vi "SUB_NICARD_DTMF9.vi"(3 "Time Out 秒":dbl, 4 "需找到特定KEY被壓的次數":i32, 5 "Find this char":string="9", 6 "AI_Name_Receiving":string) -> (0 "Detected Numbers":string, 1 "Total Count":i32, 2 "Pass?":bool)   [LabVIEW 2011]
doc: "This example shows how to construct a simple Spectrum Analyzer example using the EASY I/O Sound VIs and the MEASUREMENT VIs. This example acquires a waveform, windows it, computes the autopower spectrum and the power and frequency of the peak frequency component. The power spectrum is graphed in the desired units."
uses:
  <vilib>/sound/lvsound.llb/Sound Format.ctl
  <vilib>/DAQmx/configure/timing.llb/DAQmx Timing (Sample Clock).vi
  <vilib>/DAQmx/create/channels.llb/DAQmx Create Channel (AI-Voltage-Basic).vi
  <vilib>/DAQmx/read.llb/DAQmx Read (Analog 1D DBL 1Chan NSamp).vi
  <vilib>/Analysis/NI_AALPro.lvlib
panel:
  out "error out":errorcluster
  out "Begin Time":u32
  in  "clear":bool
  out "high tone":dbl
  out "low tone":dbl
  out "Spectrum Plot":cluster{dbl, "df":dbl, "Spectrum out":dbl[]}(graph)={0.0, "df"=10.7666015625, "Spectrum out"=[2.2239345811923915e-09, 8.683146662335903e-05, 5.401658948819699e-09, 3.283415769949573e-09, 9.087470257203412e-09, 5.196356826384313e-09, 1.0843872733561082e-08, 4.3666839571391997e-08, 7.323773949015906e-09, 2.8497866290202407e-08, 1.8346139778676557e-08, 8.325138799005256e-08, 3.709426329648907e-07, 1.0144554155621068e-07, 1.4859985315839882e-08, 2.4076563517443918e-08, 1.3199122618695927e-08, 3.4089918312362413e-07, 3.6647748653227776e-08, 2.1872311499262826e-07, 8.686470585259585e-07, 1.3633533191204446e-06, 1.809178172260895e-06, 6.207150699649024e-07, 1.88584897213167e-06, 9.53443075462152e-07, 8.595628778203373e-06, 1.6534093489189502e-05, 8.565381366748433e-06, 3.934368638186503e-06, 2.673398134714082e-06, 7.620166221013746e-07, 2.018558207269129e-06, 2.445724570769696e-05, 4.90872869304964e-06, 1.2172709001598665e-05, 9.405478455395956e-06, 1.6026544209442022e-05, 3.1157695023137614e-05, 0.00010045066273845566, 0.00010099562444668703, 0.00010789070486165799, 1.915813665106557e-05, 1.0487977511963416e-05, 7.094885886145816e-05, 3.322502717803691e-05, 3.175752599123204e-06, 6.984547958898752e-06, 8.122003278929465e-05, 7.657590620424026e-05, 6.720711760531132e-05, 0.00027943324712291083, 1.9805707230316307e-05, 4.50827477517238e-05, 6.0571130135876217e-05, 0.00021856285906605584, 0.00038709341896675954, 0.0002252713059067297, 0.00013722927061328232, 0.00025744130739904097, 0.00031585831536121644, 0.00028812421894327536, 8.629231121040524e-05, 0.00019142781529715328, 0.0017885090818483191, 0.004444937101978304, 0.002747724841296513, 0.00011579632868297775, 0.0013646075587948122, 0.0035542620245009146, 0.001429284269391688, 4.9135884119093836e-05, 0.00010438991046028727, 0.0002092766335322915, 0.0005706029316243163, 0.0011927099686592443, 0.002202098299693849, 0.0042447756964313806, 0.002184938955182395, 0.0013931881329623834, 0.000611791345491331, 0.00014384098592416903, 0.002089648172238157, 0.0014604892491541625, 0.001672902813259857, 0.0020996846985977796, 0.0018267042820125684, 0.00024143153807025544, 0.002728954825480649, 0.00016124193611955143, 0.007491288639908926, 0.01608076261438152, 0.0076505026127518016, 0.0009127306549049931, 0.00011906946681760085, 0.0006340416871388245, 0.0007338175758111943, 2.5182502508708624e-06, 0.0014774150320969704, 0.0034280107997651014, 0.004065940033575572, 0.0001807139654879104, 0.0015134026443213385, 0.0011456998362453944, 0.00010824998720249853, 0.002948833243774608, 0.00012048947131529409, 0.0032335488260886737, 0.003226548109806722, 4.90267994721965e-05, 0.00069147886170929, 5.666823215140518e-05, 0.0005823192819762041, 0.0009022477028271505, 0.0005517533787869191, 0.0003117207285129016, 0.0003908753871750581, 0.0001541062450876749, 0.00039676777157499044, 0.00021195970391491326, 2.6234631508778257e-05, 0.0002658837847014447, 0.00036345197596954665, 0.0003636016946459504, 0.0002883525548514524, 0.0002323997797870554, 0.00045117546603606835, 0.0007831715089129511, 0.00037697969403779224, 0.00025684169148288533, 0.00010464265607880238, 0.00015392030920770804, 0.000571268118545142, 0.0001791281135008112, 1.82407915272795e-05, 1.3435216977496377e-05, 6.613286083519268e-05, 6.85306300694302e-05, 3.106260409346511e-05, 7.043306599712916e-05, 7.446350251160272e-05, 7.807453839697811e-05, 4.641495088994314e-05, 4.594124976757755e-06, 2.6361087556609282e-05, 5.408410897184997e-05, 4.840864204869872e-05, 3.0852881930333154e-05, 1.4632960335315108e-05, 7.27125525658015e-05, 0.0001295923092952229, 8.06079297415985e-05, 1.2892262186773693e-05, 3.912635943158275e-05, 0.00018875463470383673, 0.00046239539279871813, 9.83461014422302e-05, 0.00010431991121427508, 5.7426568744302205e-05, 1.2919647585699225e-05, 1.3333446843951983e-05, 8.00557455545567e-05, 0.0002140654846038062, 0.00018799784777159107, 8.297670421251171e-05, 3.356795673514294e-05, 9.249862040099823e-06, 2.9018278924853506e-07, 4.5754135907992884e-05, 5.226444686010533e-05, 1.3393528265419317e-05, 5.861689249679998e-06, 6.754517491150961e-05, 0.00025201542605521695, 0.00012663622684922263, 8.354734534008234e-05, 9.900401690907939e-05, 1.0203246067824091e-05, 1.3846422437959727e-05, 1.7513782918600468e-05, 2.2531470225547707e-05, 3.570026999460579e-05, 5.608394459352944e-06, 3.5507984663188685e-08, 6.193650127282948e-06, 5.485683901026815e-06, 4.893254891786411e-05, 5.752391322110518e-05, 3.500417190819705e-05, 3.491426035627687e-05, 1.2227919637292493e-05, 9.326738918780702e-05, 0.00012903483454479285, 0.00011419716448848833, 8.886505769204026e-05, 2.9281175535596163e-05, 8.132081786205703e-06, 8.97985862152433e-07, 4.8247392248735155e-05, 5.367945684187481e-05, 3.633225820245703e-05, 9.022031345501884e-06, 2.0929305851300513e-05, 6.752089148961767e-06, 3.286214637706205e-06, 3.6662630198477625e-07, 7.763291731476242e-07, 1.3399945907103394e-06, 5.085966555258911e-06, 1.077887668545493e-05, 1.1281582963565783e-05, 1.155397820681578e-05, 4.6520974337610276e-05, 2.3309391421773472e-05, 6.845693658632664e-06, 2.704122544346558e-06, 6.665125665645291e-06, 1.0876441922754335e-05, 5.608797346818875e-06, 8.296695137818328e-07, 2.03813752326054e-06, 1.0973914063981042e-05, 1.9892910350080524e-05, 4.191121605107763e-06, 1.808715991023127e-06, 9.795606447014282e-06, 9.022632252180524e-06, 2.2366113182871527e-06, 1.436223524998135e-05, 5.7260934078321705e-06, 4.825080996478945e-06, 2.1388562191637884e-05, 1.763101781807734e-05, 2.2587628529471817e-06, 1.983067720399453e-07, 3.909338538260015e-07, 4.5350273020466913e-07, 8.343654577854134e-06, 6.790839886647775e-06, 2.255636327297339e-06, 2.584488445117655e-06, 6.824174854821624e-08, 1.372661787015302e-06, 7.194056251356914e-06, 4.541157254321738e-06, 1.6303668540732263e-06, 8.110116936046172e-07, 9.818519159870482e-07, 6.537064705721577e-07, 6.165130865665045e-07, 6.814246977481835e-07, 5.142784956191243e-06, 1.2862670435653503e-06, 3.431212791692102e-06, 6.717152893884229e-07, 5.0793672092905424e-06, 5.091843002358143e-06, 3.3788601899426006e-06, 1.6294942179365793e-06, 3.2052888551651294e-06, 2.505011537891627e-06, 1.8986099392174936e-06, 8.895175541066118e-07, 1.3175069598051258e-06, 4.119412961373611e-06, 1.7694268293659887e-06, 4.6245139735427074e-07, 4.085574744081603e-06, 6.641800395694785e-06, 2.3866053854954935e-07, 6.7501963295773596e-06, 1.3861042484181615e-05, 3.691970172195625e-06, 3.9272846697908543e-07, 3.1694989865639504e-07, 2.201281939330297e-06, 1.9502880819500733e-06, 9.578342900676284e-07, 3.83131360027214e-08, 1.9515784635010561e-07, 2.9878004194019836e-06, 4.081752511669434e-06, 7.209641153264918e-07, 8.693458519441707e-08, 4.6824501323622113e-08, 1.6560973862183618e-07, 2.0079696309823287e-07, 2.1630743971307335e-06, 2.23361594841029e-06, 3.166336475982508e-08, 1.419563103629219e-06, 3.0006577783992975e-06, 2.124654816469341e-06, 4.1221962384799796e-07, 1.4312683542199081e-06, 1.7737127563135207e-06, 9.697151883610893e-07, 7.954478190626394e-07, 1.1992527144472837e-06, 8.855607963063999e-07, 1.6461066449965424e-07, 1.7397212300863859e-07, 8.556536030808307e-07, 1.353353790123818e-07, 9.394460603994867e-07, 1.4424479309137508e-07, 1.6772776914222815e-07, 7.247702472793038e-07, 1.9063669000254936e-06, 1.887443849495326e-06, 1.8925707210222315e-06, 1.0040375911083587e-06, 7.552902303940092e-07, 1.8020303869132393e-06, 1.0587142496314781e-06, 1.459031411847178e-06, 1.4347870788937637e-06, 2.0172474849463537e-06, 1.516022898250378e-06, 3.2596374238585613e-07, 2.1549499015163616e-07, 2.586117511547747e-06, 1.8362715158444338e-06, 1.3581697014034016e-06, 9.715110917820086e-07, 2.2519613957274757e-08, 8.046610762626154e-07, 1.1130490891085315e-06, 1.3216986457543798e-07, 8.016611790474239e-07, 7.954966525566603e-07, 3.287552824052373e-07, 3.1999251102532676e-07, 1.9773782303361322e-06, 7.57049324561171e-07, 2.899671781808912e-07, 1.9745982550542387e-06, 1.4817821073364632e-06, 4.2207281783042705e-07, 2.859510597989451e-06, 6.65169327673545e-07, 1.3108579688597603e-06, 1.9279525632742265e-06, 1.923607859494516e-06, 3.7608877809167786e-07, 8.770605149941596e-08, 1.4085300538439131e-06, 1.2665811768763722e-06, 1.8672220783028666e-07, 1.6249157461690274e-06, 3.0133475481236383e-07, 6.955888433270435e-07, 1.4486995359594106e-06, 1.19907829055927e-06, 9.753115535094555e-07, 4.6454715494736343e-07, 2.454857073207436e-06, 5.444677191663221e-06, 3.151266111199155e-06, 2.0365010021356476e-06, 3.763692357617005e-07, 2.8048385043293254e-07, 7.267621498153388e-07, 1.897445548683447e-06, 9.801545193276826e-07, 5.034122710723187e-07, 8.546959157775001e-07, 5.726282029332936e-08, 1.790518893028658e-07, 1.619379081284686e-07, 1.6374366581195436e-06, 2.2925538126773367e-06, 4.1761747260056753e-07, 3.958797175774531e-07, 7.972425726207277e-07, 3.4033204403124756e-07, 1.940413284776906e-06, 7.47966836993988e-08, 1.4378795743103673e-06, 8.471793410934394e-07, 4.6447241003195404e-07, 1.6666364624086332e-07, 6.184453795459414e-08, 1.038190704797001e-07, 6.865153388263582e-07, 5.491932744056226e-07, 7.736989677920619e-08, 4.874378562302079e-07, 3.00965029667906e-07, 5.423676481238429e-07, 6.72738762673129e-07, 5.018387553252361e-07, 1.4247024148982255e-06, 3.4300270666082203e-07, 1.6301756163139806e-06, 1.8215300880149825e-06, 1.0797103355618773e-07, 1.9041653191023335e-07, 7.743539027667847e-07, 4.534623961465652e-07, 2.2330057360512448e-07, 3.132811548231781e-07, 1.022133188486526e-06, 6.274155220759265e-07, 6.903427238780778e-07, 7.33567481947441e-07, 2.047023910845942e-07, 2.791277398928224e-07, 1.3222939038823352e-06, 1.2382074249353341e-06, 3.0602357137379264e-08, 3.226519226595554e-07, 1.4358933700160236e-07, 2.161999598210508e-07, 7.226405438923372e-07, 7.82781403633883e-07, 1.406298955204302e-06, 1.2978368125295453e-06, 1.0787385566291683e-06, 7.74693414922409e-07, 1.0280376744316506e-07, 1.897257118504827e-07, 4.0674154164735285e-07, 3.3330924842068594e-07, 5.647220323383419e-07, 1.3067977141464316e-07, 6.21291802684579e-08, 6.959387220834736e-08, 2.978875001494869e-08, 1.1417698207989842e-08, 1.1088891892277042e-06, 2.1693278042962233e-06, 1.3106423009701006e-06, 9.751035000237095e-07, 3.9079154946663974e-07, 1.9665634688411184e-07, 8.019395828747413e-08, 5.648358376218229e-07, 8.755518865790549e-07, 2.1544487475681563e-07, 8.997104969411794e-08, 2.6406756196946574e-07, 9.499330882404733e-07, 4.6505226539756276e-07, 1.683265150296703e-07, 1.9973962216810128e-07, 4.5604784891804473e-07, 1.0038766206556954e-07, 1.2139267125159811e-08, 3.600082456137448e-08, 6.456671217308024e-08, 4.5206944177849573e-08, 5.120895166543777e-07, 5.020703551538299e-07, 1.4358445110590547e-08, 1.087422035023867e-07, 2.904937040652121e-07, 9.965912368812135e-08, 1.567195405704097e-07, 3.607977162533612e-07, 8.661286097636492e-07, 2.0043494023967716e-07, 1.404349876871561e-08, 1.155747877697829e-08, 8.948817141186363e-08, 5.8027285180593554e-08, 4.073116484984666e-08, 1.3308592777960855e-07, 2.3957183564679474e-08, 6.957435335895439e-08, 6.155244039483246e-08, 2.4444043310448568e-08, 2.670800778057559e-08, 5.7216353702400666e-08, 9.239854415332251e-08, 3.0213042230580236e-08, 1.343191141960498e-09, 2.0837817399160295e-08, 2.602661931976853e-08, 6.8560172643748795e-09, 7.916856835570337e-08, 9.00267241744782e-08, 7.692528448413547e-08, 1.2004889715129119e-08, 9.88727747790812e-08, 1.0023405452613187e-07, 1.210633991600998e-07, 2.1522628537105935e-08, 5.6078990716154034e-08, 5.4328268985728565e-08, 7.382864407910501e-08, 3.0003386035033976e-08, 1.2666181215774758e-07, 1.447357694076088e-08, 4.5027939045110415e-08, 5.3269947199899464e-08, 3.859299030969913e-08, 3.241786088144045e-08, 2.720065882503426e-09, 1.2643450599208627e-08, 1.964613447417824e-07, 2.0620303225395736e-07, 3.960659464702874e-08, 5.470531246980156e-08, 2.1669113140794644e-08, 3.908095826759173e-09, 2.49346348700968e-09, 6.457620819587205e-08, 7.514895182622606e-08, 9.756339699497464e-09, 6.350841154899524e-09, 1.2441504257846113e-07, 2.140824153645837e-07, 7.93683699567381e-08, 2.9681442249265694e-08, 1.0955395323608218e-08, 4.758727775105736e-08, 3.1114217067159584e-08, 2.8431649831268218e-08, 7.886529468547796e-08, 6.928095914063998e-08, 6.44062797559934e-08, 1.5729337740057154e-07, 1.633584064839165e-07, 3.805955578821095e-08, 3.4997453344192845e-08, 8.022151382112027e-08, 8.574249753493645e-08, 8.12990606975002e-08, 1.9694836264953252e-08, 1.0791818303309123e-08, 1.570533231452924e-08, 7.382425248896943e-10, 3.9250377730515e-08, 4.72955171147271e-08, 8.090028033459793e-08, 1.0325474748498492e-07, 5.1119681074873145e-08, 7.094343264085443e-08, 2.9392859253071123e-08, 9.238628151896506e-09, 5.694530625648633e-08, 1.8625727600349932e-07, 3.322703462873384e-08, 3.425440210880957e-08, 3.4277236525869975e-08, 3.617970164543665e-08, 1.4707673577394132e-08, 1.2922454182753588e-10, 1.8095931082295038e-08, 5.600407565406485e-09, 8.953513148727372e-09, 2.3611851256797674e-08, 1.146166540157641e-08, 2.201964779928675e-08, 2.9764039172426437e-08, 2.961234359885526e-08, 5.5575454720846034e-08, 1.590716964180081e-08, 2.5499378001220853e-08, 8.486556471190526e-09, 4.204027722433145e-09, 1.0654218030939125e-08, 5.474455330294607e-08, 5.4653270431217174e-08, 4.783079993275118e-08, 4.6046354336983404e-08, 7.990893299542365e-09, 2.3198558294294397e-08, 2.9547812456393353e-08, 1.2653880062427829e-08, 1.7251579240159026e-08, 4.63416262611152e-08, 1.5129601159503794e-08, 2.3139266486687776e-09, 1.828690977536453e-08, 2.2861672881711013e-08, 3.8144074954067966e-08, 2.8840406985371016e-08, 1.1468655141246242e-08, 1.6179157979919108e-08, 2.9612534185614193e-08, 4.232564980227527e-08, 5.807228261326083e-09, 1.193918664246388e-08, 9.555146125407209e-09, 2.6756709498907878e-08, 3.5854514290437304e-08, 3.3536922761277736e-08, 1.6236282954676824e-08, 1.419182533462672e-08, 1.8960043424887072e-08, 2.2529888699703793e-08, 2.769640618611182e-08, 1.7752768144773262e-08, 3.817051129247205e-08, 3.9146068301267074e-08, 2.701166800566469e-08, 3.6083532480292083e-08, 4.759826701599105e-08, 2.2528709606772587e-08, 1.4373847425932876e-08, 1.0108916334457278e-08, 4.344209392987958e-09, 2.76248817252588e-09, 3.345855814497143e-08, 3.1876958273761295e-08, 1.0309771452695787e-08, 7.480054719232873e-09, 6.934965945389653e-09, 1.021958155170289e-08, 4.726637225820998e-09, 2.7923791885579298e-08, 2.615594662610562e-09, 5.685726703733775e-10, 6.436791353396253e-09, 3.971859921789547e-09, 5.451134199864811e-09, 5.599761079275237e-09, 1.8091294273463573e-09, 6.459132929182603e-09, 5.657936238218396e-09, 1.950038474358936e-08, 3.902896651024208e-08, 2.6647511591608208e-08, 1.7167991854833567e-08, 5.705082172612073e-09, 1.1906878405088487e-09, 6.430332981144355e-10, 3.044261872785727e-10, 5.40091869318323e-09, 1.145469490858611e-08, 4.512515382960901e-09, 1.268872354479999e-09, 8.69571281338811e-11, 5.979719362973721e-09, 8.303067196362185e-09, 1.039890454681567e-09, 4.403612351010871e-09, 6.1893486406988e-09, 3.744143658237287e-09, 1.6098151770992428e-09, 5.248990067906987e-10, 8.470755606628997e-09, 7.463249915147587e-09, 1.0295767797537241e-09, 3.4956972619547825e-09, 5.641606872154712e-09, 4.994213570996723e-10, 2.405446245720403e-09, 1.489678532464873e-09, 2.2902032474967982e-10, 1.8935576252770074e-09, 6.140797401991911e-09, 4.138757232522736e-09, 1.4205243196923323e-08, 1.0122644492215224e-08, 1.0308696632691912e-09, 3.7261704680704176e-09, 2.219667711519674e-09, 1.5818367931203758e-10, 3.1956703588648097e-10, 3.728028330933628e-09, 5.204819070783557e-09, 2.3182128777113778e-09, 5.54274237431268e-09, 5.912467923961738e-09, 3.4984304800838524e-10, 1.7519583360697777e-09, 3.5760658885376834e-09, 2.920707192498906e-09, 4.991604442354138e-09, 5.22047326033885e-09, 1.1121882980094295e-08, 1.0515997862901546e-08, 8.56222533176954e-09, 2.16240545488912e-09, 3.4438501798671816e-10, 1.8304744483799816e-09, 7.928375487876729e-09, 5.625674085292935e-09, 2.599916438756517e-09, 3.5181591731768393e-09, 2.1217829342968287e-09, 2.2753003599648508e-09, 3.4226665411631988e-09, 5.636839365927383e-09, 7.482358015828702e-09, 3.4894051216861324e-09, 5.081541309898216e-10, 5.232121738196756e-10, 3.4140952661333457e-09, 5.535791400541489e-09, 2.330868115515569e-09, 7.282566020209013e-10, 7.872180714469127e-10, 2.0937186224820734e-09, 4.385762477016771e-09, 4.662321859562959e-09, 1.0936849727646788e-09, 1.779919440059085e-09, 5.814676588780071e-10, 1.4243028963503696e-09, 7.711594786984741e-09, 3.529621264712184e-09, 2.676389419868003e-09, 4.024900708447496e-09, 8.979532033775118e-10, 1.387096810631821e-09, 6.16168707641335e-10, 1.3043500724006639e-09, 1.0060661688154498e-09, 5.272350241092032e-10, 4.842385157592935e-10, 4.79401273594476e-09, 5.555714769211231e-09, 3.071678971190096e-09, 4.256573526238938e-09, 1.928446419086416e-09, 4.416159046828467e-10, 3.767639009725344e-09, 2.952303872960992e-09, 1.7643182268094367e-09, 1.184159894053597e-09, 2.7932934526917684e-09, 1.9368817963660564e-09, 2.7430528754171613e-09, 5.225587432169088e-10, 3.203199932968183e-10, 1.9797615162730513e-09, 8.560689437790192e-10, 1.3756570831157762e-09, 2.077805905489259e-09, 3.53465334234968e-09, 4.860234675895279e-09, 2.124017257302096e-09, 5.853203456602198e-11, 2.516050984534377e-09, 7.880997614550843e-10, 7.37630554137802e-10, 7.31937655708805e-10, 7.602633332778057e-10, 1.4973872311600496e-10, 2.832501177732104e-09, 3.4088527208373545e-09, 2.10419737941665e-09, 1.7856704137105817e-09, 1.8829909904485974e-09, 1.6885012672101362e-11, 9.981932083310103e-11, 4.923391793317421e-10, 5.488431723286112e-10, 3.1535776708464555e-11, 1.2576645527152945e-10, 3.195193563516089e-11, 2.9010054595514423e-11, 5.3959324436706067e-11, 4.207578635912359e-10, 1.3434752942557352e-09, 8.388553690154514e-10, 3.709413955497562e-10, 2.310126954666965e-11, 1.9412886393254603e-10, 1.5256275616250847e-09, 1.2700530378170274e-09, 1.0145820142699707e-09, 9.02812894090267e-11, 2.380865008764687e-10, 1.3884639791549605e-10, 7.097231542592393e-10, 1.4705312317889802e-10, 3.862728542670797e-10, 6.164191610984895e-10, 2.660938261830858e-10, 4.1980202338370243e-10, 4.174891700935234e-10, 1.9551068467012963e-10, 1.2809251895251019e-09, 1.2010818631768713e-09, 8.023763127102151e-10, 2.301277278510448e-10, 2.282367771403777e-10, 2.802656534310578e-10, 2.8381567604717416e-09, 1.3056140440628833e-09, 9.946000302107385e-10, 2.019650934949039e-10, 6.17402391077043e-11, 5.067315270594634e-10, 8.495763773619358e-11, 7.685765214095721e-12, 6.596099326938714e-11, 1.5977878807757865e-10, 1.3505898652283798e-10, 3.2339161959433536e-10, 9.181248445894812e-10, 9.033526336502124e-10, 9.365426508084887e-11, 1.5835643049796864e-09, 1.109253745919973e-09, 4.743298781860182e-10, 3.987212410725e-12, 9.016453427310602e-11, 2.2564563875148533e-10, 2.170213485823025e-10, 2.4632504239019264e-11, 8.685537809384159e-10, 5.0716890250874e-10, 8.171582894823122e-13, 1.2319527875084226e-10, 2.794878076018828e-10, 1.9098550224368597e-10, 2.243856772517594e-10, 3.721139454800636e-10, 7.543450869519107e-11, 5.492907359358165e-10, 7.441572939818098e-10, 5.563714854922252e-10, 2.3442621156495966e-10, 7.122534088655344e-12, 5.438935026364515e-11, 3.058752272772633e-11, 7.964657206284309e-11, 1.322930734820325e-10, 4.1828035722374734e-10, 4.825514587076015e-10, 2.3601908260282152e-11, 9.995037669671284e-11, 2.8837286106756752e-11, 7.7584161635509e-11, 4.925186582086759e-11, 4.3123223628482706e-11, 6.001348439876205e-11, 2.660823203179512e-10, 5.835097679116502e-11, 2.4371074101681597e-12, 2.8708263655531525e-10, 1.0452331220034235e-10, 1.7419411308588767e-11, 1.586938787690648e-11, 2.614011077415245e-10, 1.906391801272774e-10, 8.608172097402236e-10, 6.359406235781075e-10, 9.55087274351948e-11, 7.420039646561873e-10, 4.277854440466337e-10, 2.514884199120615e-10, 1.87362909024348e-10, 5.816583664209649e-12, 3.0748210371688494e-11, 1.1617001225093083e-10, 1.543372698055287e-10, 2.1164907244552623e-11, 1.5339034521507372e-10, 1.1296774574948826e-10, 3.545703672449203e-10, 6.838348267836377e-11, 2.666691344937961e-10, 4.01146646127394e-12, 2.8253853309552043e-11, 4.865860582627764e-11, 3.812971990283942e-11, 3.513905009113374e-10, 7.262049749655285e-11, 2.7076218803863766e-10, 1.679038424025831e-10, 1.191512488410735e-10, 1.6762637771545003e-10, 1.1570677133729292e-10, 2.93701692757346e-11, 8.985694145300448e-11, 5.378560526480976e-12, 1.5111522532685182e-11, 9.33784088613121e-12, 8.108969569702798e-11, 7.344604239441166e-11, 2.749158285282731e-11, 1.149440726370342e-10, 7.558184550049066e-11, 1.0388688445068887e-10, 2.3884411611108205e-11, 4.523702881859529e-11, 5.539444652117604e-11, 1.2505846602408144e-10, 1.391237889983128e-10, 1.0229838641777619e-10, 2.2760448461751894e-10, 1.6878930272235683e-11, 5.563133519338542e-11, 2.4795564168072182e-11, 4.88300841319007e-12, 2.753076326726938e-10, 5.0745585442639115e-11, 1.9748881750443707e-11, 4.7253681970740655e-11, 1.1828022584495795e-12, 6.307397956109176e-11, 1.2112903811280616e-11, 3.7736829220246094e-11, 1.2666717771535954e-11, 9.110131621536755e-12, 1.4356147174808164e-10, 4.835735472117299e-11, 1.6119503703271416e-10, 2.7284220732102933e-11, 6.252917322874483e-11, 4.3224534315473703e-11, 1.0498695216758215e-10, 1.974346778432821e-11, 5.40782337396056e-11, 5.2369100478518394e-11, 2.2326679398260537e-12, 1.3443392922630235e-10, 1.5137082145318955e-11, 7.602967117655898e-11, 1.6705324428778388e-12, 8.087034464306943e-11, 2.843203593917431e-11, 4.3869855642256153e-11, 9.094608127233439e-12, 5.1610906648717704e-11, 4.5769346158818275e-11, 8.91014346500043e-12, 2.1390251716311653e-11, 6.369147522118072e-11, 2.0219657267618414e-11, 7.614932077706351e-11, 8.380130770612789e-14, 7.44685721218674e-11, 4.889713918700368e-12, 2.8824435687798222e-11, 2.336178035548185e-11, 2.032069895529248e-11, 3.177186397825414e-11, 1.829839515856845e-11, 1.7199587674909958e-11, 2.3830341916764486e-11, 3.936674241530467e-11, 1.4530112344764962e-11, 6.42340167219902e-11, 6.543850560478522e-12, 3.180552492573337e-11, 2.640733156400162e-11, 2.3998816474733135e-11, 1.4707500600098032e-11, 2.2677492907918244e-11, 2.5488024985826562e-11, 2.2847423539048195e-11, 2.6508742451231927e-11, 2.7455219413636878e-11, 1.9014114797814238e-11, 1.4498235090545703e-11, 2.971065931438831e-11, 2.8238743649172455e-11, 1.5558166743438014e-11, 1.5480415800015573e-11, 2.743925897718036e-11, 2.7495492280695883e-11, 9.799113867949333e-12, 3.6747692894834385e-11, 8.199934716177243e-12, 4.0755373799372346e-11, 2.121428785076837e-11, 1.5541949260482237e-11, 2.798920514032833e-11, 1.7462178669667912e-11, 2.344077180370279e-11, 1.3268735286972787e-11, 3.290786429192333e-11, 1.3582414980189854e-11, 2.1254639689841874e-11, 3.125190775410135e-11, 1.1594584974728011e-11, 2.0766725629006086e-11, 2.5397224688363225e-11, 2.017197976315566e-11, 2.1560267022375116e-11, 1.8478426377320472e-11, 2.185880297981598e-11, 2.3207271921244853e-11, 1.6644091551449067e-11, 2.5159531873055792e-11, 1.7387326911492145e-11, 2.2342088396302478e-11, 1.878186953930171e-11, 2.1386854408980777e-11, 1.6296384472522648e-11, 2.665785605014739e-11, 1.932225503661904e-11, 1.7990103900180257e-11, 2.280409760981406e-11, 2.0876076757621922e-11, 1.6705840903949015e-11, 2.447838243286913e-11, 1.9386127278251222e-11, 1.9972810505022722e-11, 2.094081228451663e-11, 2.089112317638976e-11, 1.8529128535041152e-11, 2.1003285317481698e-11, 2.1626975006946126e-11, 1.959173405923362e-11, 1.9951310126412882e-11, 2.056616361421096e-11, 2.0129355353149965e-11, 2.081460915369522e-11, 1.9548428298641114e-11, 2.099219771829391e-11, 1.969977451051827e-11, 2.0914920833116317e-11, 1.976452612506575e-11, 2.061186299405415e-11, 1.994600938714932e-11, 2.0573926789305875e-11, 1.9999209922834507e-11, 2.0465454689399724e-11, 2.0178494817701738e-11, 2.0384946662937728e-11, 2.0181301433592506e-11, 2.0287338520900114e-11, 2.028072242449754e-11, 2.0263007390114753e-11, 2.0273179004249868e-11]}
  # "Settings"
  # "Detected Tones"
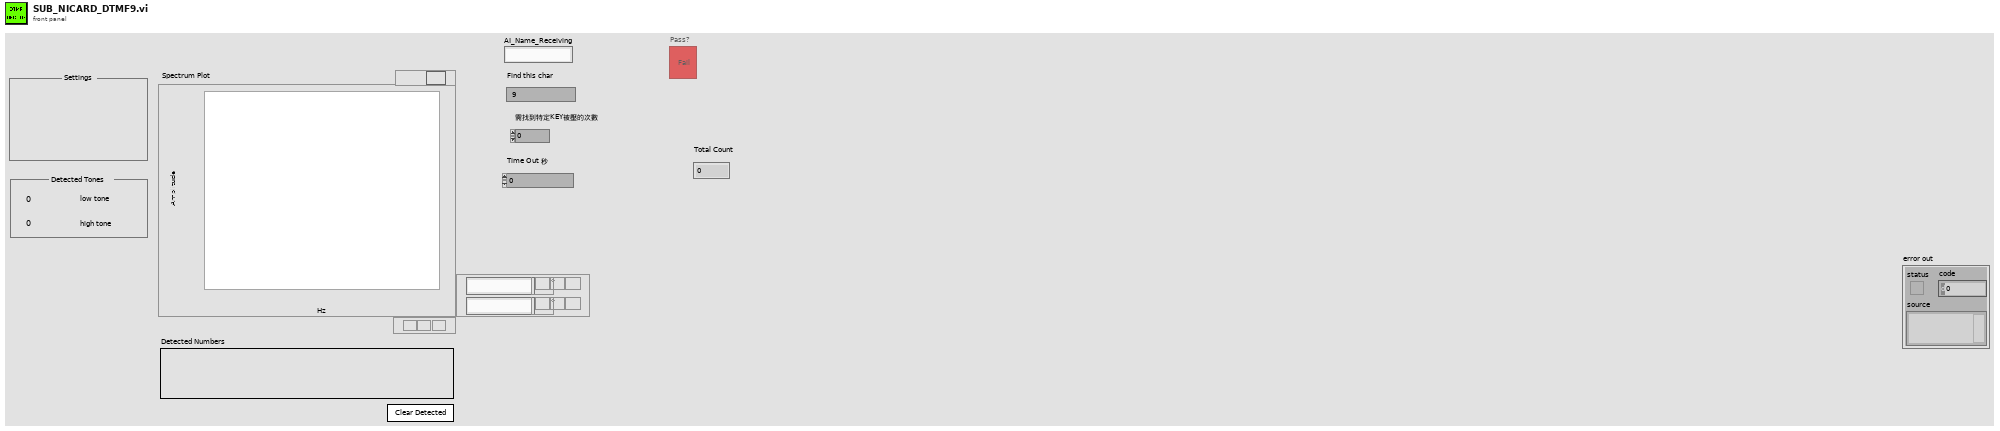
[diagram p1: front panel]
types:
  T1 = typedef "Sound Format.ctl" = cluster{"sound quality":enum16{"mono", "stereo"}, "rate":enum16{"11025", "22050", "44100", "8000"}, "bits per sample":enum16{"8 bit", "16 bit"}}
  T2 = enum32{"Lowpass", "Highpass", "Bandpass", "Bandstop"}
  T3 = cluster{dbl, "df":dbl, "Power Spectrum (V^2 rms)":dbl[]}
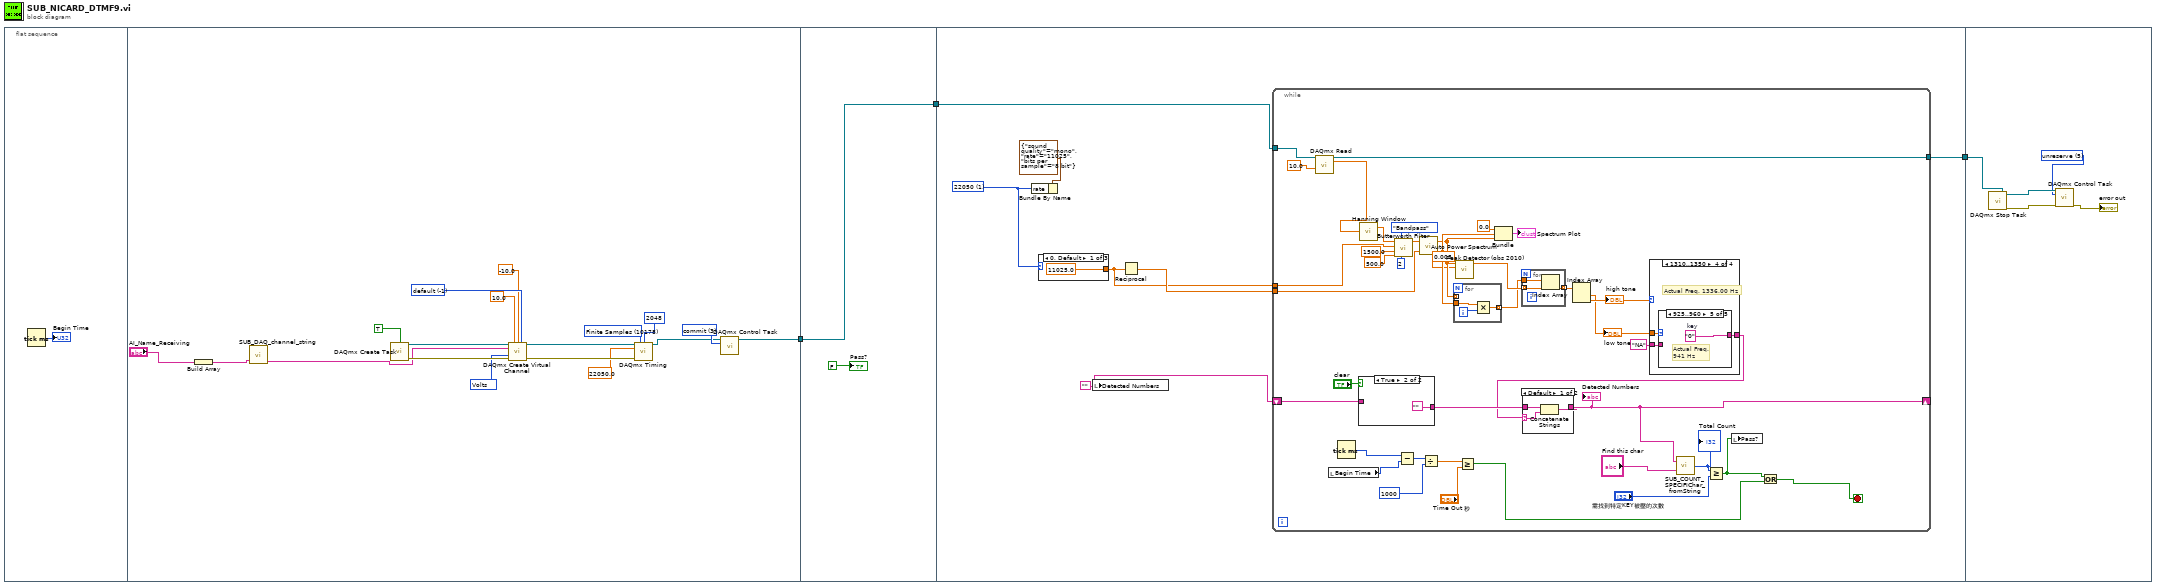
[diagram p0: block diagram]
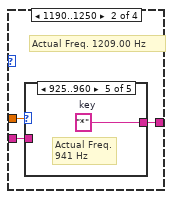
[diagram p5: hidden frame]
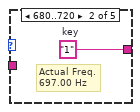
[diagram p7: hidden frame]
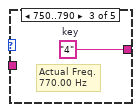
[diagram p8: hidden frame]
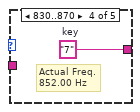
[diagram p9: hidden frame]
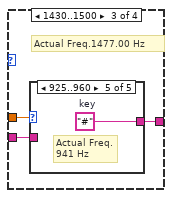
[diagram p10: hidden frame]
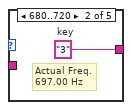
[diagram p12: hidden frame]
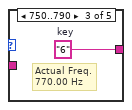
[diagram p13: hidden frame]
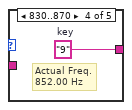
[diagram p14: hidden frame]
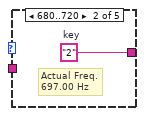
[diagram p16: hidden frame]
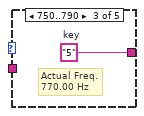
[diagram p17: hidden frame]
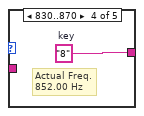
[diagram p18: hidden frame]
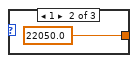
[diagram p19: hidden frame]
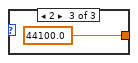
[diagram p20: hidden frame]
diagram:
  n1 = flat-sequence {
    tunnel: [w5] -> w2
    tunnel: [w23] -> w3
    tunnel: w2 -> [w23]
    tunnel: w3 -> [w26]
    tunnel: [w25] -> w1
    tunnel: w1 -> [w112]
    frame #0 {
      n2 = Tick Count (ms)() -> (millisecond timer value=→"Begin Time":u32)
    }
    frame #1 {
      w8 = -1 items=["default"=-1, "RSE"=10083, "NRSE"=10078, "Differential"=10106, "Pseudodifferential"=12529] ("input terminal configuration")
      w12 = 10348 items=["Volts"=10348, "From Custom Scale"=10065] ("units")
      w15 = 3 items=["verify"=2, "reserve"=4, "commit"=3, "unreserve"=5, "abort"=6] ("action")
      w17 = 10178 items=["Finite Samples"=10178, "Continuous Samples"=10123, "Hardware Timed Single Point"=12522] ("sample mode")
      n3 = Build Array("AI_Name_Receiving") -> (w9:string[])
      n4 = call "SUB_DAQ_channel_string.vi"("channel"=w9) -> ("resulting string"=w11:string)  [unwired: 1 in, 2 out]
      n5 = call <vilib>:"DAQmx Create Task.vi"("auto cleanup"=TRUE) -> ("task out"=w21:refnum<k21>, "error out"=w20:errorcluster)  [unwired: 13 in]
      n6 = call-poly <vilib>:"DAQmx Create Virtual Channel.vi"("task in"=w21, "maximum value"=10.0, "minimum value"=-10.0, "input terminal configuration"=w8, "physical channels"=w11, "units"=w12, "error in"=w20) -> ("task out"=w14:refnum<k21>, "error out"=w19:errorcluster)  [unwired: 7 in]
      n7 = call-poly <vilib>:"DAQmx Timing.vi"("task/channels in"=w14, "sample mode"=w17, "samples per channel"=2048, "rate"=22050.0, "error in"=w19) -> ("task out"=w13:refnum<k21>)  [unwired: 9 in, 1 out]
      n8 = call <vilib>:"DAQmx Control Task.vi"("task/channels in"=w13, "action"=w15) -> ("task out"=w5:refnum<k21>)  [unwired: 12 in, 1 out]
    }
    frame #2 {
      "Pass?" <- FALSE
    }
    frame #3 {
      w31 = u16 1 items=["11025", "22050", "44100"] ("Sample Rate")
      w27 = ""
      n9 = Bundle By Name(cluster=T1 {"sound quality"=enum."mono", "rate"=enum."11025", "bits per sample"=enum."8 bit"} ("sound format"), "rate"=w31) -> ()  [unwired: 1 out]
      n10 = case shown="0, Default" w31 {
        tunnel: [11025.0 22050.0 44100.0] -> w28
        frame 0, Default {
        }
        frame 1 {
        }
        frame 2 {
        }
      }
      n11 = local write "Detected Numbers"(w27) -> ()
      n12 = Reciprocal(x=w28) -> (1/x=w29:dbl)
      n13 = while {
        tunnel: w29 -> [w70]
        tunnel: w28 -> [w60]
        shift-right: [w48] -> _
        shift-left: w27 -> [w51]
        tunnel: w26 -> [w33]
        tunnel: [w32] -> w25
        stop <- w36 stop-if-true
        n14 = call-poly <vilib>:"DAQmx Read.vi"("task/channels in"=w33, "timeout"=10.0) -> ("task out"=w32:refnum<k21>, "data"=w34:dbl[])  [unwired: 11 in, 1 out]
        n15 = local read "Begin Time"() -> (w38:u32)
        n16 = Tick Count (ms)() -> (millisecond timer value=w37:u32)
        n17 = case shown="True" "clear" {
          tunnel: [w72 ""] -> w52
          tunnel: w51 -> [w72 _]
          frame False {
          }
          frame True {
          }
        }
        n18 = call "Hanning Window.vi"("X"=w34) -> ("Hanning {X}"=w61:dbl[])  [unwired: 1 out]
        n19 = call "Butterworth Filter.vi"("order"=2, "filter type"=T2."Bandpass", "low cutoff freq: fl"=500.0, "high cutoff freq: fh"=1500.0, "sampling freq: fs"=w60, "X"=w61) -> ("Filtered X"=w67:dbl[])  [unwired: 2 in, 1 out]
        n20 = Subtract(x=w37, y=w38) -> (x-y=w44:u32)
        n21 = call "Auto Power Spectrum.vi"("dt"=w70, "Signal (V)"=w67) -> ("df"=w56:dbl, "Power Spectrum (V^2 rms)"=w55:dbl[])
        n22 = Divide(x=w44, y=u32 1000) -> (x/y=w42:dbl)
        n23 = for {
          tunnel: w56 -> [w104]
          tunnel: [w103] -> w65 mode=indexing
          tunnel: w55 -> [_] mode=indexing
          i -> [w105]
          n24 = Multiply(x=w104, y=w105) -> (x*y=w103:dbl)
        }
        n25 = call <vilib>:"Peak Detector (obs 2010).vi"("threshold"=0.005 ("Detection Threshold"), "X"=w55) -> ("Locations"=w66:dbl[])  [unwired: 5 in, 4 out]
        n26 = Greater Or Equal?(x=w42, y="Time Out 秒") -> (x >= y?=w39:bool)
        n27 = Bundle(0.0, "df"=w56, "Power Spectrum (V^2 rms)"=w55) -> (→"Spectrum Plot":T3)  [unwired: 1 in]
        n28 = for {
          tunnel: w66 -> [w107] mode=indexing
          tunnel: w65 -> [w108]
          tunnel: [w106] -> w64 mode=indexing
          n29 = Index Array(array=w108, index=w107) -> (element=w106:dbl)
        }
        n30 = Index Array(array=w64) -> (element #1=w58:dbl, element #2=w59:dbl)  [unwired: 2 in]
        "low tone" <- w58
        "high tone" <- w59
        n31 = case shown="1310..1350" w59 {
          tunnel: w58 -> [_ w81 w89 w97]
          tunnel: [w78 w80 w88 w96] -> w49
          tunnel: "NA" ("Button") -> [w78 w79 w87 w95]
          frame Default {
          }
          frame 1190..1250 {
            # "Actual Freq. 1209.00 Hz"
            n32 = case shown="925..960" w81 {
              tunnel: [w82 w83 w84 w85 w86] -> w80
              tunnel: w79 -> [w82 _ _ _ _]
              frame Default {
              }
              frame 680..720 {
                w83 = "1"  # key
                # "Actual Freq. 697.00 Hz"
              }
              frame 750..790 {
                w84 = "4"  # key
                # "Actual Freq. 770.00 Hz"
              }
              frame 830..870 {
                w85 = "7"  # key
                # "Actual Freq. 852.00 Hz"
              }
              frame 925..960 {
                w86 = "*"  # key
                # "Actual Freq. 941 Hz"
              }
            }
          }
          frame 1430..1500 {
            # "Actual Freq.1477.00 Hz"
            n33 = case shown="925..960" w89 {
              tunnel: [w90 w91 w92 w93 w94] -> w88
              tunnel: w87 -> [w90 _ _ _ _]
              frame Default {
              }
              frame 680..720 {
                w91 = "3"  # key
                # "Actual Freq. 697.00 Hz"
              }
              frame 750..790 {
                w92 = "6"  # key
                # "Actual Freq. 770.00 Hz"
              }
              frame 830..870 {
                w93 = "9"  # key
                # "Actual Freq. 852.00 Hz"
              }
              frame 925..960 {
                w94 = "#"  # key
                # "Actual Freq. 941 Hz"
              }
            }
          }
          frame 1310..1350 {
            # "Actual Freq. 1336.00 Hz"
            n34 = case shown="925..960" w97 {
              tunnel: [w98 w99 w100 w101 w102] -> w96
              tunnel: w95 -> [w98 _ _ _ _]
              frame Default {
              }
              frame 680..720 {
                w99 = "2"  # key
                # "Actual Freq. 697.00 Hz"
              }
              frame 750..790 {
                w100 = "5"  # key
                # "Actual Freq. 770.00 Hz"
              }
              frame 830..870 {
                w101 = "8"  # key
                # "Actual Freq. 852.00 Hz"
              }
              frame 925..960 {
                w102 = "0"  # key
                # "Actual Freq. 941 Hz"
              }
            }
          }
        }
        n35 = case shown="Default" w49 {
          selector: w49 -> [w74 _]
          tunnel: w52 -> [w76 w77]
          tunnel: [w75 w77] -> w48
          frame Default {
            n36 = Concatenate Strings(w76, w74) -> (w75:string)
          }
          frame "NA" {
          }
        }
        "Detected Numbers" <- w48
        n37 = call "SUB_COUNT_SPECIFIChar_fromString.vi"("Find this char"="Find this char", "Input String"=w48) -> ("Total Count"=w46:i32)
        "Total Count" <- w46
        n38 = Greater Or Equal?(x=w46, y="需找到特定KEY被壓的次數") -> (x >= y?=w40:bool)
        n39 = local write "Pass?"(w40) -> ()
        n40 = Or(x=w40, y=w39) -> (x .or. y?=w36:bool)
      }
    }
    frame #4 {
      w114 = 5 items=["verify"=2, "reserve"=4, "commit"=3, "unreserve"=5, "abort"=6] ("action")
      n41 = call <vilib>:"DAQmx Stop Task.vi"("task/channels in"=w112) -> ("task out"=w116:refnum<k21>, "error out"=w115:errorcluster)  [unwired: 13 in]
      n42 = call <vilib>:"DAQmx Control Task.vi"("task/channels in"=w116, "action"=w114, "error in"=w115) -> ("error out"=→"error out":errorcluster)  [unwired: 11 in, 1 out]
    }
  }
